vi "HEWH Index Data.vi"(7 "Basic Index?":bool, 8 "error in (no error)":errorcluster, 9 "Data Index Location":i32, 10 "Test Data-Start to End DBL":dbl[][](array[numeric]), 11 "Draw Index":i32[](array[numeric])) -> (0 "error out":errorcluster, 2 "Basic Index Output":dbl, 3 "Extracted Data":dbl[](array[numeric]))   [LabVIEW 2023]
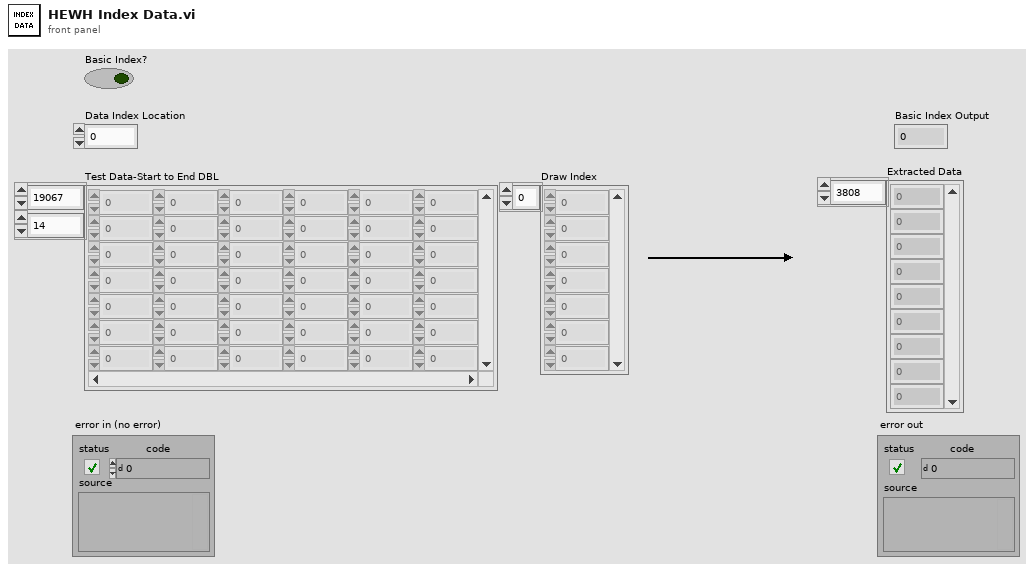
[diagram p1: front panel]
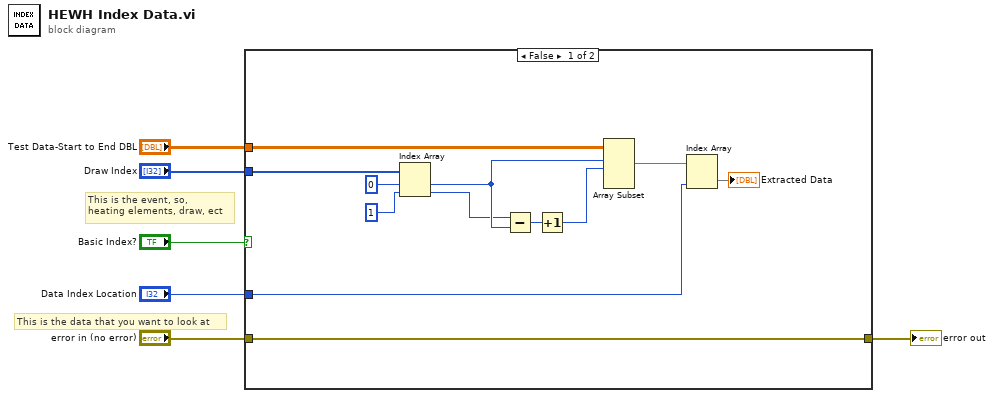
[diagram p0: block diagram]
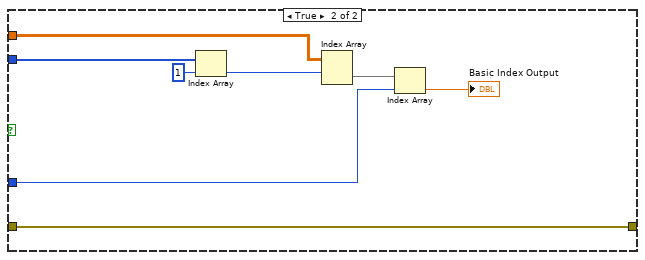
[diagram p2: hidden frame]
diagram:
  # "This is the event, so,\nheating elements, draw, ect"
  # "This is the data that you want to look at"
  n1 = case shown="False" "Basic Index?" {
    tunnel: "Data Index Location" -> [w8 w20]
    tunnel: "Test Data-Start to End DBL" -> [w9 w22]
    tunnel: "Draw Index" -> [w10 w21]
    tunnel: "error in (no error)" -> [w11 w26]
    tunnel: [w11 w26] -> w2
    frame False {
      n2 = Index Array "Index Array"(array=w10, index #1=0 ("index"), index #2=1 ("index")) -> (element #1=w17:i32, element #2=w13:i32)
      n3 = Subtract(x=w13, y=w17) -> (x-y=w12:i32)
      n4 = Increment(x=w12) -> (x+1=w7:i32)
      n5 = Array Subset "Array Subset"(array=w9, index (row)=w17, length (row)=w7) -> (w16:dbl[][])  [unwired: 2 in]
      n6 = Index Array "Index Array"(array=w16, index (col)=w8) -> (element=→"Extracted Data":dbl[])  [unwired: 1 in]
    }
    frame True {
      n7 = Index Array "Index Array"(array=w21, index=1) -> (element=w24:i32)
      n8 = Index Array "Index Array"(array=w22, index (row)=w24) -> (element=w25:dbl[])  [unwired: 1 in]
      n9 = Index Array "Index Array"(array=w25, index=w20) -> (element=→"Basic Index Output":dbl)
    }
  }
  "error out" <- w2
